vi "Facade.vi"(0 "Data In":T4, 2 "Display State In":T2={"format string"="%#_g", "font size"=13, "invalid text"="<Auto>", "valid range"={"min"=-inf, "max"=0.0}, "size"={"width"=100, "height"=22}, "numeric text color"=0, "overlay text color"=6553600}, 3 "Container State":T3) -> (6 "Data Out":T4, 7 "Display State Out":T2={"format string"="%#_g", "font size"=13, "invalid text"="<Auto>", "valid range"={"min"=-inf, "max"=0.0}, "size"={"width"=100, "height"=22}, "numeric text color"=0, "overlay text color"=6553600}, 8 "Action":T1)   [LabVIEW 2017, in "Numeric with String Overlay.xctl"]
uses:
  <vilib>/addons/_XControls/Numeric with String Overlay/Numeric with String Overlay.xctl
  <vilib>/addons/_XControls/Numeric with String Overlay/Data.ctl
  <vilib>/_xctls/Container State.ctl
  <vilib>/addons/_XControls/Numeric with String Overlay/State.ctl
  <vilib>/_xctls/Action.ctl
  <vilib>/Utility/miscctls.llb/LVMenuShortCut.ctl
  <vilib>/Utility/miscctls.llb/LVBoundsTypeDef.ctl
  <vilib>/_xctls/XControlSupport.lvlib
panel:
  out "string":string
  in  "numeric":dbl caption="Data"
  in  "skin":string
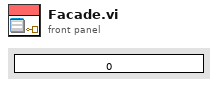
[diagram p1: front panel]
types:
  T1 = typedef "XControlSupport.lvlib/Action.ctl" = cluster{"Data Changed?":bool, "State Changed?":bool, "Action Name":string}
  T2 = typedef "Numeric with String Overlay.xctl/State.ctl" = cluster{"format string":string, "font size":u32, "invalid text":string, "valid range":cluster{"min":dbl, "max":dbl}, "size":cluster{"width":u32, "height":u32}, "numeric text color":u32, "overlay text color":u32}
  T3 = typedef "XControlSupport.lvlib/Container State.ctl" = cluster{"Indicator?":bool, "Run Mode?":bool, " Refnum":refnum<vi>}
  T4 = typedef "Numeric with String Overlay.xctl/Data.ctl" = dbl
  T5 = typedef "LVMenuShortCut.ctl" = cluster{"Include Shift Key?":bool, "Include Ctrl Key?":bool, "Shortcut Key":string}
  T6 = typedef "LVBoundsTypeDef.ctl" = cluster{"Width":u32, "Height":u32}
  T7 = typedef "LVPositionTypeDef.ctl" = cluster{"Left":i32, "Top":i32}
  T8 = typedef "LVRectTypeDef.ctl" = cluster{"Left":i16, "Top":i16, "Right":i16, "Bottom":i16}
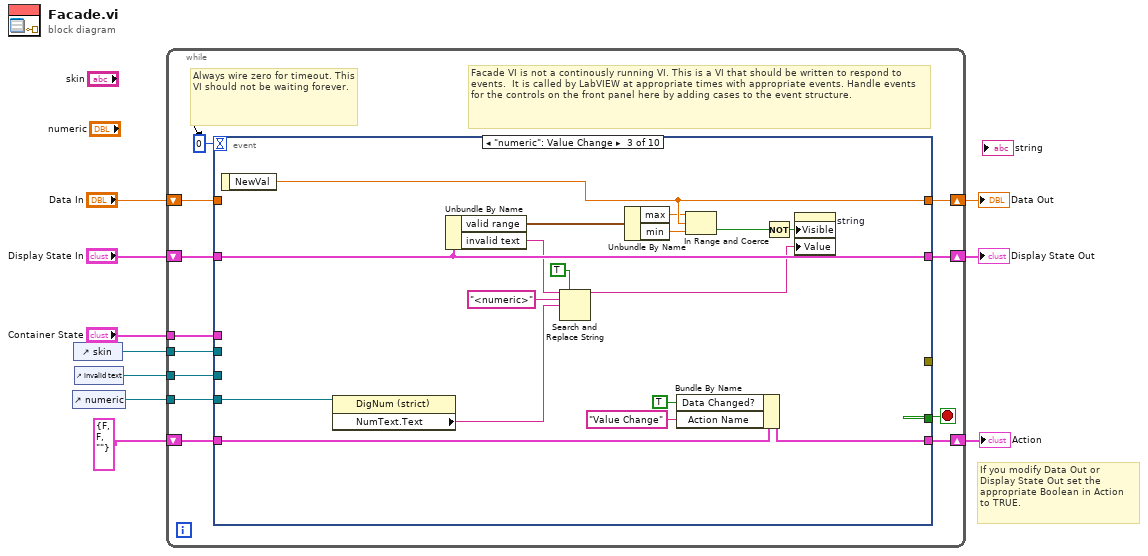
[diagram p0: block diagram]
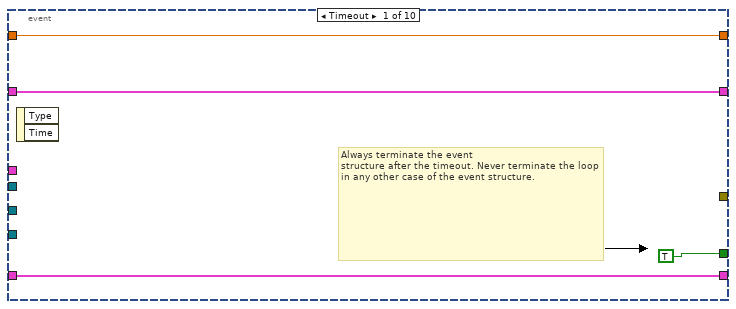
[diagram p2: hidden frame]
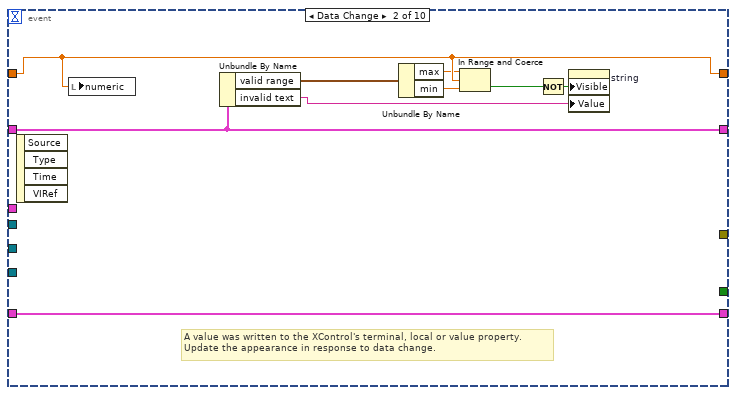
[diagram p3: hidden frame]
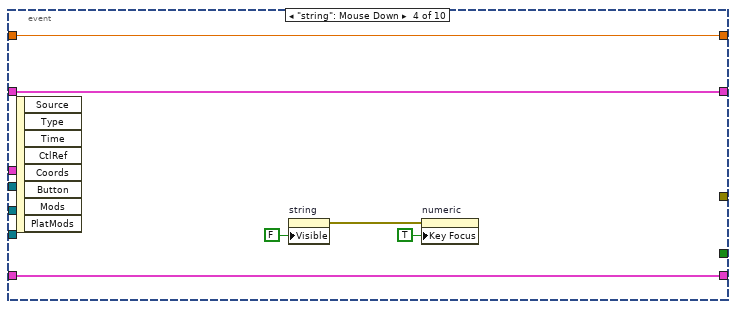
[diagram p4: hidden frame]
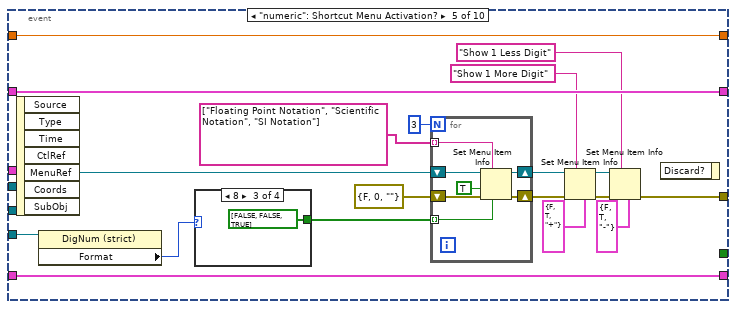
[diagram p5: hidden frame]
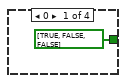
[diagram p6: hidden frame]
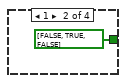
[diagram p7: hidden frame]
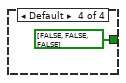
[diagram p8: hidden frame]
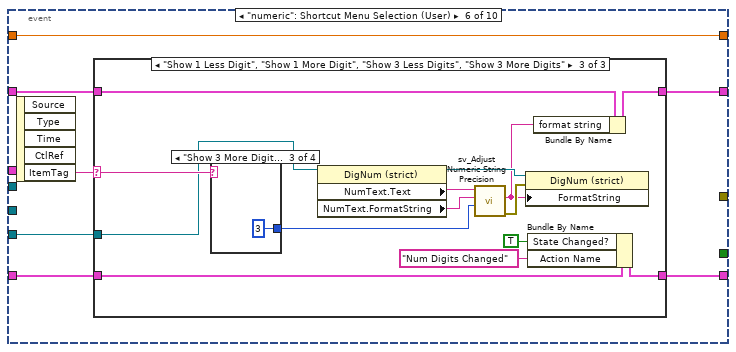
[diagram p9: hidden frame]
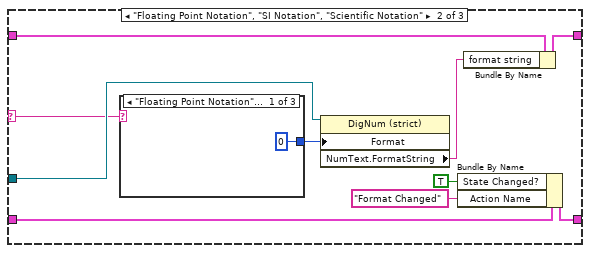
[diagram p11: hidden frame]
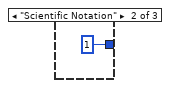
[diagram p12: hidden frame]
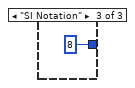
[diagram p13: hidden frame]
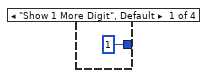
[diagram p14: hidden frame]
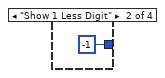
[diagram p15: hidden frame]
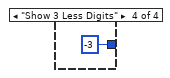
[diagram p16: hidden frame]
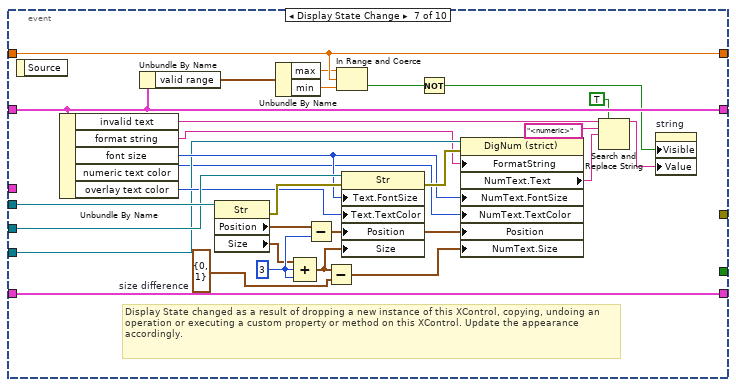
[diagram p17: hidden frame]
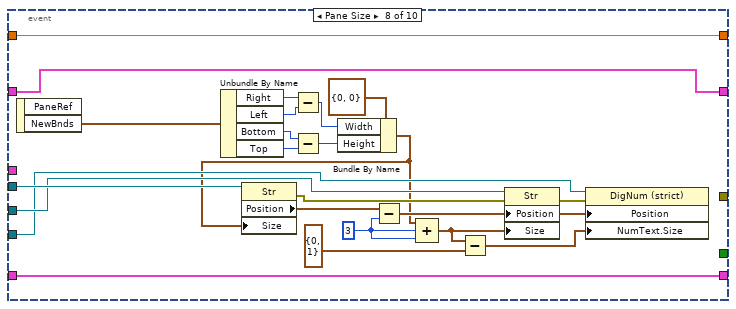
[diagram p18: hidden frame]
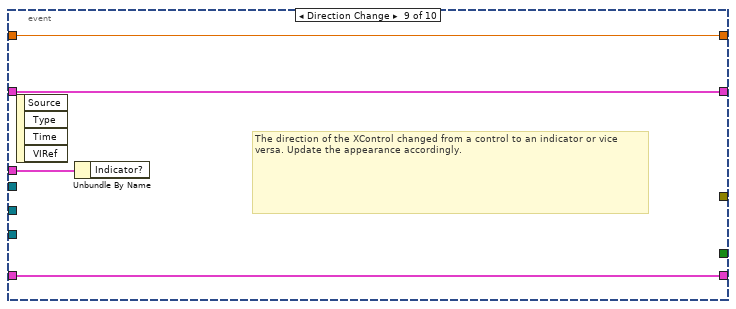
[diagram p19: hidden frame]
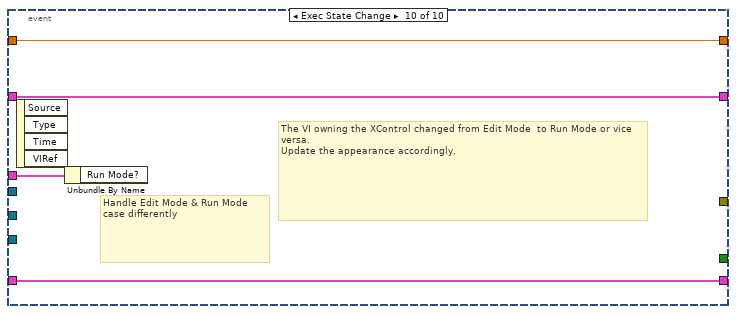
[diagram p20: hidden frame]
diagram:
  # "If you modify Data Out or\nDisplay State Out set the\nappropriate Boolean in Action\nto TRUE."
  n1 = control-ref of="numeric"() -> (w1:refnum<vi>)
  n2 = control-ref of="skin"() -> (w3:refnum<vi>)
  n3 = control-ref of="invalid text"() -> (w2:refnum<vi>)
  n4 = while {
    shift-right: [w21] -> w7
    shift-left: "Display State In" -> [w22]
    tunnel: "Container State" -> [w18]
    shift-right: [w16] -> w10
    shift-left: "Data In" -> [w17]
    shift-right: [w14] -> w5
    shift-left: T1 {"Data Changed?"=FALSE, "State Changed?"=FALSE, "Action Name"=""} ("Action") -> [w15]
    tunnel: w3 -> [w13]
    tunnel: w2 -> [w12]
    tunnel: w1 -> [w11]
    stop <- w20 stop-if-true
    # "Facade VI is not a continously running VI. This is a VI that should be written to respond to events.  It is called by LabVIEW at appropriate times with appropriate events. Handle events for the controls on the front panel here by adding cases to the event structure."
    # "Always wire zero for timeout. This\nVI should not be waiting forever."
    n5 = event shown="[2] \"numeric\": Value Change" {
      selector: _ -> [_ _ _ _ _ _ _ _ _ _]
      dyn-events: _ -> [_ _ _ _ _ _ _ _ _ _]
      timeout: 0 -> [_ _ _ _ _ _ _ _ _ _]
      tunnel: w22 -> [w24 w31 w52 w58 w77 w92 w148 w159 w183 w187]
      tunnel: [w24 w31 w52 w58 w77 w91 w148 w159 w183 w187] -> w21
      tunnel: [TRUE _ _ _ _ _ _ _ _ _] -> w20
      tunnel: w18 -> [_ _ _ _ _ _ _ _ w184 w188]
      tunnel: w17 -> [w23 w29 _ w57 w76 w95 w134 w180 w182 w186]
      tunnel: [w23 w29 w44 w57 w76 w95 w134 w180 w182 w186] -> w16
      tunnel: [w25 w35 w47 w56 w75 w89 w157 w179 w181 w185] -> w14
      tunnel: w15 -> [w25 w35 w48 w56 w75 w90 w157 w179 w181 w185]
      tunnel: w13 -> [_ _ _ _ _ _ w156 w173 _ _]
      tunnel: w12 -> [_ _ _ _ _ _ w155 w172 _ _]
      tunnel: w11 -> [_ _ w42 _ w71 w94 w140 w162 _ _]
      tunnel: [_ _ _ _ w61 _ _ _ _ _] -> _
      event Timeout {
        # "Always terminate the event\nstructure after the timeout. Never terminate the loop in any other case of the event structure."
        n6 = event-data() -> ()  [unwired: 1 in, 2 out]
      }
      event Data Change {
        # "A value was written to the XControl's terminal, local or value property.\nUpdate the appearance in response to data change."
        n7 = event-data() -> ()  [unwired: 1 in, 4 out]
        n8 = local write "numeric"(w29) -> ()
        n9 = Unbundle By Name(w31) -> ("valid range"=w34:cluster{"min":dbl, "max":dbl}, "invalid text"=w30:string)
        n10 = Unbundle By Name(w34) -> ("max"=w28:dbl, "min"=w27:dbl)
        n11 = In Range and Coerce(upper limit=w28, x=w29, lower limit=w27) -> (In Range?=w33:bool)  [unwired: 1 out]
        n12 = Not(x=w33) -> (.not. x?=w32:bool)
        n13 = property on="string" class="Str"("Visible"=w32, "Value"=w30) -> ()  [unwired: 2 in, 2 out]
      }
      event "numeric": Value Change {
        n14 = event-data() -> ("NewVal"=w44:dbl)  [unwired: 1 in]
        n15 = property class="DigNum (strict)"(reference=w42) -> ("NumText.Text"=w41:string)  [unwired: 1 in, 2 out]
        n16 = Unbundle By Name(w52) -> ("valid range"=w51:cluster{"min":dbl, "max":dbl}, "invalid text"=w40:string)
        n17 = Search and Replace String(replace all?=TRUE ("replace all? (F)"), input string=w40, search string="<numeric>", replace string=w41) -> (result string=w39:string)  [unwired: 4 in, 3 out]
        n18 = Unbundle By Name(w51) -> ("max"=w37:dbl, "min"=w36:dbl)
        n19 = Bundle By Name(cluster=w48, "Data Changed?"=TRUE, "Action Name"="Value Change") -> (w47:T1)
        n20 = In Range and Coerce(upper limit=w37, x=w44, lower limit=w36) -> (In Range?=w50:bool)  [unwired: 1 out]
        n21 = Not(x=w50) -> (.not. x?=w49:bool)
        n22 = property on="string" class="Str"("Visible"=w49, "Value"=w39) -> ()  [unwired: 2 in, 2 out]
      }
      event "string": Mouse Down {
        n23 = event-data() -> ()  [unwired: 1 in, 8 out]
        n24 = property on="string" class="Str"("Visible"=FALSE) -> (error out=w53:errorcluster)  [unwired: 2 in, 1 out]
        n25 = property on="numeric" class="DigNum (strict)"(error in=w53, "Key Focus"=TRUE) -> ()  [unwired: 1 in, 2 out]
      }
      event "numeric": Shortcut Menu Activation? {
        n26 = event-data() -> ("MenuRef"=w74:refnum<k9>)  [unwired: 1 in, 6 out]
        n27 = property class="DigNum (strict)"(reference=w71) -> ("Format"=w70:u8)  [unwired: 1 in, 2 out]
        n28 = case shown="8" w70 {
          tunnel: [bool[] [TRUE, FALSE, FALSE] bool[] [FALSE, TRUE, FALSE] bool[] [FALSE, FALSE, TRUE] bool[] [FALSE, FALSE, FALSE]] -> w69
          frame 0 {
          }
          frame 1 {
          }
          frame 8 {
          }
          frame Default {
          }
        }
        n29 = for {
          N: 3 -> [_]
          tunnel: string[] ["Floating Point Notation", "Scientific Notation", "SI Notation"] -> [w87] mode=indexing
          tunnel: w69 -> [w86] mode=indexing
          shift-right: [w84] -> w68
          shift-left: w74 -> [w88]
          shift-right: [w83] -> w60
          shift-left: errorcluster {"status"=FALSE, "code"=0, "source"=""} ("error out") -> [w82]
          n30 = Set Menu Item Info(6:w86, 7:w87, 8:w82, 9:TRUE ("enabled"), 11:w88) -> (0:w83:errorcluster, 3:w84:refnum<k9>)  [unwired: 2 in]
        }
        n31 = Set Menu Item Info(4:T5 {"Include Shift Key?"=FALSE, "Include Ctrl Key?"=TRUE, "Shortcut Key"="+"} ("short cut"), 7:"Show 1 More Digit" ("item tag"), 8:w60, 11:w68) -> (0:w65:errorcluster, 3:w64:refnum<k9>)  [unwired: 3 in]
        n32 = Set Menu Item Info(4:T5 {"Include Shift Key?"=FALSE, "Include Ctrl Key?"=TRUE, "Shortcut Key"="-"} ("short cut"), 7:"Show 1 Less Digit" ("item tag"), 8:w65, 11:w64) -> (0:w61:errorcluster)  [unwired: 3 in, 1 out]
        n33 = event-data() -> ()  [unwired: 2 in, 1 out]
      }
      event "numeric": Shortcut Menu Selection (User) {
        n34 = event-data() -> ("ItemTag"=w93:string)  [unwired: 1 in, 4 out]
        n35 = case shown="\"Show 1 Less Digit\", \"Show 1 More Digit\", \"Show 3 Less Digits\", \"Show 3 More Digits\"" w93 {
          selector: w93 -> [_ w106 w124]
          tunnel: w94 -> [_ w107 w121]
          tunnel: w92 -> [w97 w104 w117]
          tunnel: [w97 w103 w116] -> w91
          tunnel: w90 -> [w96 w101 w114]
          tunnel: [w96 w100 w111] -> w89
          frame Default {
          }
          frame "Floating Point Notation", "SI Notation", "Scientific Notation" {
            n36 = case shown="\"Floating Point Notation\", Default" w106 {
              tunnel: [u8 0 ("Display Format:Format") u8 1 ("Display Format:Format") u8 8 ("Display Format:Format")] -> w105
              frame "Floating Point Notation", Default {
              }
              frame "Scientific Notation" {
              }
              frame "SI Notation" {
              }
            }
            n37 = property class="DigNum (strict)"(reference=w107, "Format"=w105) -> ("NumText.FormatString"=w102:string)  [unwired: 1 in, 2 out]
            n38 = Bundle By Name(cluster=w101, "State Changed?"=TRUE, "Action Name"="Format Changed") -> (w100:T1)
            n39 = Bundle By Name(cluster=w104, "format string"=w102) -> (w103:T2)
          }
          frame "Show 1 Less Digit", "Show 1 More Digit", "Show 3 Less Digits", "Show 3 More Digits" {
            n40 = case shown="\"Show 3 More Digits\"" w124 {
              tunnel: [1 ("Display Format:Format") -1 ("Display Format:Format") 3 ("Display Format:Format") -3 ("Display Format:Format")] -> w119
              frame "Show 1 More Digit", Default {
              }
              frame "Show 1 Less Digit" {
              }
              frame "Show 3 More Digits" {
              }
              frame "Show 3 Less Digits" {
              }
            }
            n41 = property class="DigNum (strict)"(reference=w121) -> (reference out=w120:refnum<vi>, "NumText.Text"=w123:string, "NumText.FormatString"=w122:string)  [unwired: 1 in, 1 out]
            n42 = call <vilib>:"sv_Adjust Numeric String Precision.vi"("change in digits/precision"=w119, "original format string"=w122, "numeric text"=w123) -> ("error out"=w118:errorcluster, "new format string"=w115:string)  [unwired: 7 in]
            n43 = property class="DigNum (strict)"(reference=w120, error in=w118, "FormatString"=w115) -> ()  [unwired: 2 out]
            n44 = Bundle By Name(cluster=w114, "State Changed?"=TRUE, "Action Name"="Num Digits Changed") -> (w111:T1)
            n45 = Bundle By Name(cluster=w117, "format string"=w115) -> (w116:T2)
          }
        }
      }
      event Display State Change {
        w144 = T6 {"Width"=0, "Height"=1}  # size difference
        w153 = 3
        # "Display State changed as a result of dropping a new instance of this XControl, copying, undoing an operation or executing a custom property or method on this XControl. Update the appearance accordingly."
        n46 = event-data() -> ()  [unwired: 1 in, 1 out]
        n47 = Unbundle By Name(w148) -> ("invalid text"=w137:string, "format string"=w138:string, "font size"=w141:u32, "numeric text color"=w135:u32, "overlay text color"=w149:u32)
        n48 = Unbundle By Name(w148) -> ("valid range"=w146:cluster{"min":dbl, "max":dbl})
        n49 = property class="Str"(reference=w156) -> (error out=w151:errorcluster, "Position"=w154:T7, "Size"=w145:T6)  [unwired: 1 in, 1 out]
        n50 = Unbundle By Name(w146) -> ("max"=w130:dbl, "min"=w129:dbl)
        n51 = Compound Arithmetic op=ADD(w145, w153, w153) -> (w143:T6)
        n52 = Subtract(x=w154, y=w153) -> (x-y=w152:T7)
        n53 = Subtract(x=w143, y=w144) -> (x-y=w142:T6)
        n54 = In Range and Coerce(upper limit=w130, x=w134, lower limit=w129) -> (In Range?=w147:bool)  [unwired: 1 out]
        n55 = property class="Str"(reference=w155, error in=w151, "Text.FontSize"=w141, "Text.TextColor"=w149, "Position"=w152, "Size"=w143) -> (error out=w150:errorcluster)  [unwired: 1 out]
        n56 = Not(x=w147) -> (.not. x?=w132:bool)
        n57 = property class="DigNum (strict)"(reference=w140, error in=w150, "FormatString"=w138, "NumText.FontSize"=w141, "NumText.TextColor"=w135, "Position"=w152, "NumText.Size"=w142) -> ("NumText.Text"=w136:string)  [unwired: 2 out]
        n58 = Search and Replace String(replace all?=TRUE ("replace all? (F)"), input string=w137, search string="<numeric>", replace string=w136) -> (result string=w131:string)  [unwired: 4 in, 3 out]
        n59 = property on="string" class="Str"("Visible"=w132, "Value"=w131) -> ()  [unwired: 2 in, 2 out]
      }
      event Pane Size {
        w177 = 3
        n60 = event-data() -> ("NewBnds"=w171:T8)  [unwired: 1 in, 1 out]
        n61 = Unbundle By Name(w171) -> ("Right"=w170:i16, "Left"=w169:i16, "Bottom"=w168:i16, "Top"=w167:i16)
        n62 = Subtract(x=w170, y=w169) -> (x-y=w165:i16)
        n63 = Subtract(x=w168, y=w167) -> (x-y=w164:i16)
        n64 = Bundle By Name(cluster=T6 {"Width"=0, "Height"=0} ("Size"), "Width"=w165, "Height"=w164) -> (w158:T6)
        n65 = property class="Str"(reference=w173, "Size"=w158) -> (error out=w175:errorcluster, "Position"=w178:T7)  [unwired: 1 in, 1 out]
        n66 = Subtract(x=w178, y=w177) -> (x-y=w176:T7)
        n67 = Compound Arithmetic op=ADD(w158, w177, w177) -> (w160:T6)
        n68 = Subtract(x=w160, y=T6 {"Width"=0, "Height"=1}) -> (x-y=w161:T6)
        n69 = property class="Str"(reference=w172, error in=w175, "Position"=w176, "Size"=w160) -> (error out=w174:errorcluster)  [unwired: 1 out]
        n70 = property class="DigNum (strict)"(reference=w162, error in=w174, "Position"=w176, "NumText.Size"=w161) -> ()  [unwired: 2 out]
      }
      event Direction Change {
        # "The direction of the XControl changed from a control to an indicator or vice versa. Update the appearance accordingly."
        n71 = event-data() -> ()  [unwired: 1 in, 4 out]
        n72 = Unbundle By Name(w184) -> ()  [unwired: 1 out]
      }
      event Exec State Change {
        # "The VI owning the XControl changed from Edit Mode  to Run Mode or vice versa.\nUpdate the appearance accordingly."
        # "Handle Edit Mode & Run Mode\ncase differently"
        n73 = event-data() -> ()  [unwired: 1 in, 4 out]
        n74 = Unbundle By Name(w188) -> ()  [unwired: 1 out]
      }
    }
  }
  "Display State Out" <- w7
  "Data Out" <- w10
  "Action" <- w5
